vi "SelectPort.vi"() -> (0 "COM":refnum<visa-resource-name>)   [LabVIEW 2017]
panel:
  in  "OK":bool
  in  "COM Port":refnum<visa-resource-name>="COM4"
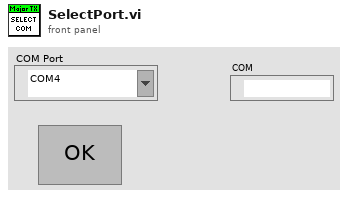
[diagram p1: front panel]
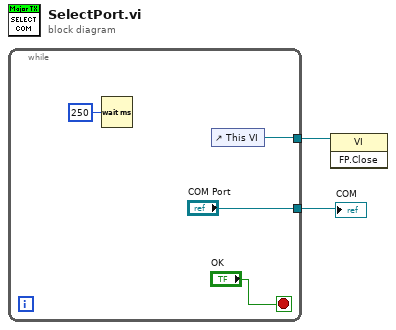
[diagram p0: block diagram]
diagram:
  n1 = while {
    tunnel: ["COM Port"] -> w1
    tunnel: [w3] -> w2
    stop <- "OK" stop-if-true
    n2 = Wait (ms)(milliseconds to wait=u32 250) -> ()  [unwired: 1 out]
    n3 = control-ref of="This VI"() -> (w3:refnum<vi>)
  }
  "COM" <- w1
  n4 = invoke class="VI" method="FP.Close"(reference=w2) -> ()  [unwired: 2 in, 3 out]
